vi "solar_type Variant Set Enum Names.vi"(7 "Enum Names":string[](array[string]), 10 "Numeric Variant (U8..U64)":variant) -> (2 "Enum Variant":variant, 5 "Enum Valid?":bool)   [LabVIEW 2018]
doc: "This sets the enum names of a numeric variant type. If an error occurs, this returns the original variant data."
uses:
  <vilib>/Utility/Data Type/NI_Data Type.lvlib
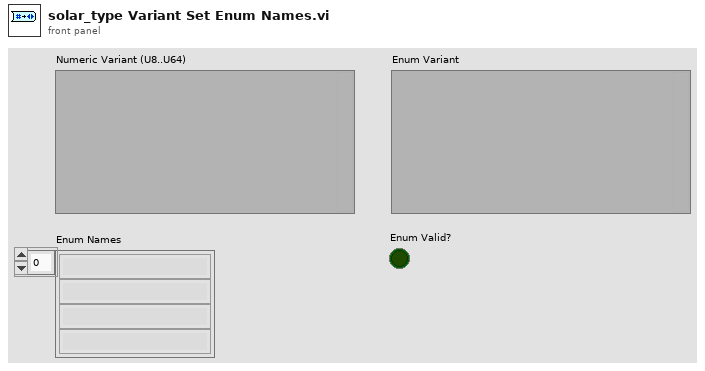
[diagram p1: front panel]
types:
  T1 = typedef "NI_Data Type.lvlib/Data Type.ctl" = enum8{"Invalid Type", "Void", "I8", "I16", "I32", "I64", "U8", "U16", "U32", "U64", "Single Float", "Double Float", "Extended Float", "Single Complex", "Double Complex", "Extended Complex", "Enum U8", "Enum U16", "Enum U32", "Enum U64", "Single Float With Unit", "Double Float With Unit", "Extended Float With Unit", "Single Complex with Unit", "Double Complex with Unit", "Extended Complex with Unit", "Boolean", "String", "Path", "Picture", "Tag", "Array", "Cluster", "Variant", "LV Variant", "Waveform", "Timestamp", "Digital Waveform", "Digital Data", "ExpressData", "Refnum", "External Data", "VI", "Poly VI", "LabVIEW Class Instance", "Fixed Point", "Set Collection", "Map Collection"}
  T2 = typedef "NI_Data Type.lvlib/Memory Info.ctl" = cluster{"Type":T3, "Size":u32}
  T3 = typedef "NI_Data Type.lvlib/Memory Type.ctl" = enum16{"Variable", "Fixed", "Bounded"}
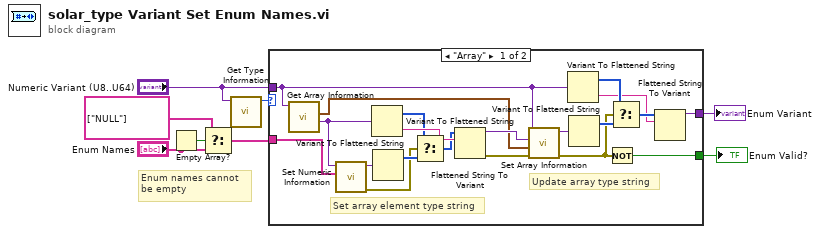
[diagram p0: block diagram]
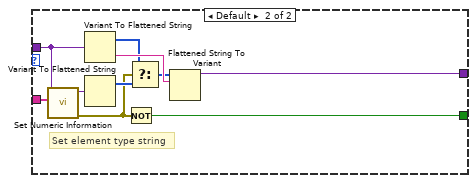
[diagram p2: hidden frame]
diagram:
  # "Enum names cannot\nbe empty"
  n1 = Empty Array?(array="Enum Names") -> (empty?=w6:bool)
  n2 = Select(t=string[] ["NULL"], s=w6, f="Enum Names") -> (s? t:f=w3:string[])
  n3 = call <vilib>:"Get Type Information.vi"("variant"="Numeric Variant (U8..U64)") -> ("type"=w1:T1)  [unwired: 6 in, 4 out]
  n4 = case shown="\"Array\"" w1 {
    tunnel: [w11 w33] -> w8
    tunnel: [w12 w31] -> w7
    tunnel: w3 -> [w10 w30]
    tunnel: "Numeric Variant (U8..U64)" -> [w15 w29]
    frame "Array" {
      # "Update array type string"
      # "Set array element type string"
      n5 = call <vilib>:"Get Array Information.vi"("variant"=w15) -> ("array element data type"=w22:variant, "array lengths"=w9:T2[])  [unwired: 7 in, 2 out]
      n6 = call <vilib>:"Set Numeric Information.vi"("Enum Names"=w10, "Variant in"=w22) -> ("error out"=w23:errorcluster, "Variant out"=w27:variant)  [unwired: 8 in]
      n7 = Variant To Flattened String(Variant=w22) -> (data string=w28:string, 1:w25:i16[])
      n8 = Variant To Flattened String(Variant=w27) -> (1:w26:i16[])  [unwired: 1 out]
      n9 = Select(t=w25, s=w23, f=w26) -> (s? t:f=w24:i16[])
      n10 = Flattened String To Variant(6:w28, 7:w24) -> (0:w20:errorcluster, 3:w21:variant)  [unwired: 1 in]
      n11 = call <vilib>:"Set Array Information.vi"("error in (no error)"=w20, "Array Lengths"=w9, "Array Element"=w21, "Variant in"=w15) -> ("error out"=w13:errorcluster, "Variant out"=w14:variant)  [unwired: 6 in]
      n12 = Variant To Flattened String(Variant=w15) -> (data string=w16:string, 1:w18:i16[])
      n13 = Variant To Flattened String(Variant=w14) -> (1:w17:i16[])  [unwired: 1 out]
      n14 = Not(x=w13) -> (.not. x?=w12:bool)
      n15 = Select(t=w18, s=w13, f=w17) -> (s? t:f=w19:i16[])
      n16 = Flattened String To Variant(6:w16, 7:w19) -> (3:w11:variant)  [unwired: 1 in, 1 out]
    }
    frame Default {
      # "Set element type string"
      n17 = call <vilib>:"Set Numeric Information.vi"("Enum Names"=w30, "Variant in"=w29) -> ("error out"=w32:errorcluster, "Variant out"=w37:variant)  [unwired: 8 in]
      n18 = Variant To Flattened String(Variant=w29) -> (data string=w38:string, 1:w35:i16[])
      n19 = Variant To Flattened String(Variant=w37) -> (1:w36:i16[])  [unwired: 1 out]
      n20 = Not(x=w32) -> (.not. x?=w31:bool)
      n21 = Select(t=w35, s=w32, f=w36) -> (s? t:f=w34:i16[])
      n22 = Flattened String To Variant(6:w38, 7:w34) -> (3:w33:variant)  [unwired: 1 in, 1 out]
    }
  }
  "Enum Variant" <- w8
  "Enum Valid?" <- w7
